vi "pmt demultiplexer control.vi"() -> ()   [LabVIEW 2017]
doc: "This example performs writes and reads on a serial port, as directed by the user. You can press the Write and Read buttons, and change the Read Count, while the example is running.\n\nThe parameters set for the serial port must match the parameters of the connected instrument or device. In this example, the Read Count parameter specifies the number of bytes that the serial port reads. If there were more bytes at the port than the specified number, those bytes would not be read. If there were less bytes at the port than the specified number, you would receive a timeout error.\n\nThis example expands upon the flow control options for XON and XOFF, allowing the user to choose those control characters. Also, the user can enable or disable a termination character. Some devices require a termination character in order to identify the end of command strings. Some devices send a termination character to signify the end of data to be read. This example shows how you can end the Read operation once a termination character is detected in the buffer and/or append a termination character at the end of the Write data."
uses:
  pmt demultiplexer command set.ctl
  <vilib>/Instr/_visa.llb/VISA Configure Serial Port (Instr).vi
panel:
  in  "encode photons as level changes":bool
  out "cross talk":dbl
  in  "dead count rate":dbl format="%#_13g"
  out "beam 2 rate":dbl
  out "beam 1 rate":dbl
  out "lock problem":bool
  in  "test input":enum8{"none", "internal", "external"}(ring)
  in  "laser cycles to veto":u8=2
  in  "start2 - start1":u16=180 step=5
  in  "width2":u16=170 max=180 step=5
  in  "width1":u16=170 max=180 step=5
  in  "auto step phase":bool
  out "version":u8[](array[numeric])
  out "cts vs phase shift":cluster{dbl[], dbl[]}[](graph)
  out "tau":dbl=0.6896638311807903
  out "dead counts":dbl=52664.79325691533
  out "exponential fit parameters":cluster{"t0":dbl, "amplitude":dbl}[](array[cluster])=[{"t0"=3.645795108508593, "amplitude"=683172.1393034825}]
  in  "timeout (ms)":i32=1000
  in  "num exp":i32=1
  out "total count rate":dbl=683172.1393034825
  out "hist data received":bool=TRUE
  out "histogram":cluster{i32[], dbl[]}[](graph)
  out "all data received":bool=TRUE
  out "response":u8[](array[numeric])
  in  "Command":T1
  in  "overall phase shift (deg)":u16=95 step=5
  out "error out":errorcluster
  in  "Stop":bool
  in  "data":u8
  in  "Send command":bool
  in  "VISA resource name":refnum<visa-resource-name>="COM8"
  # "5 deg = 200 ps @ 70 MHz"
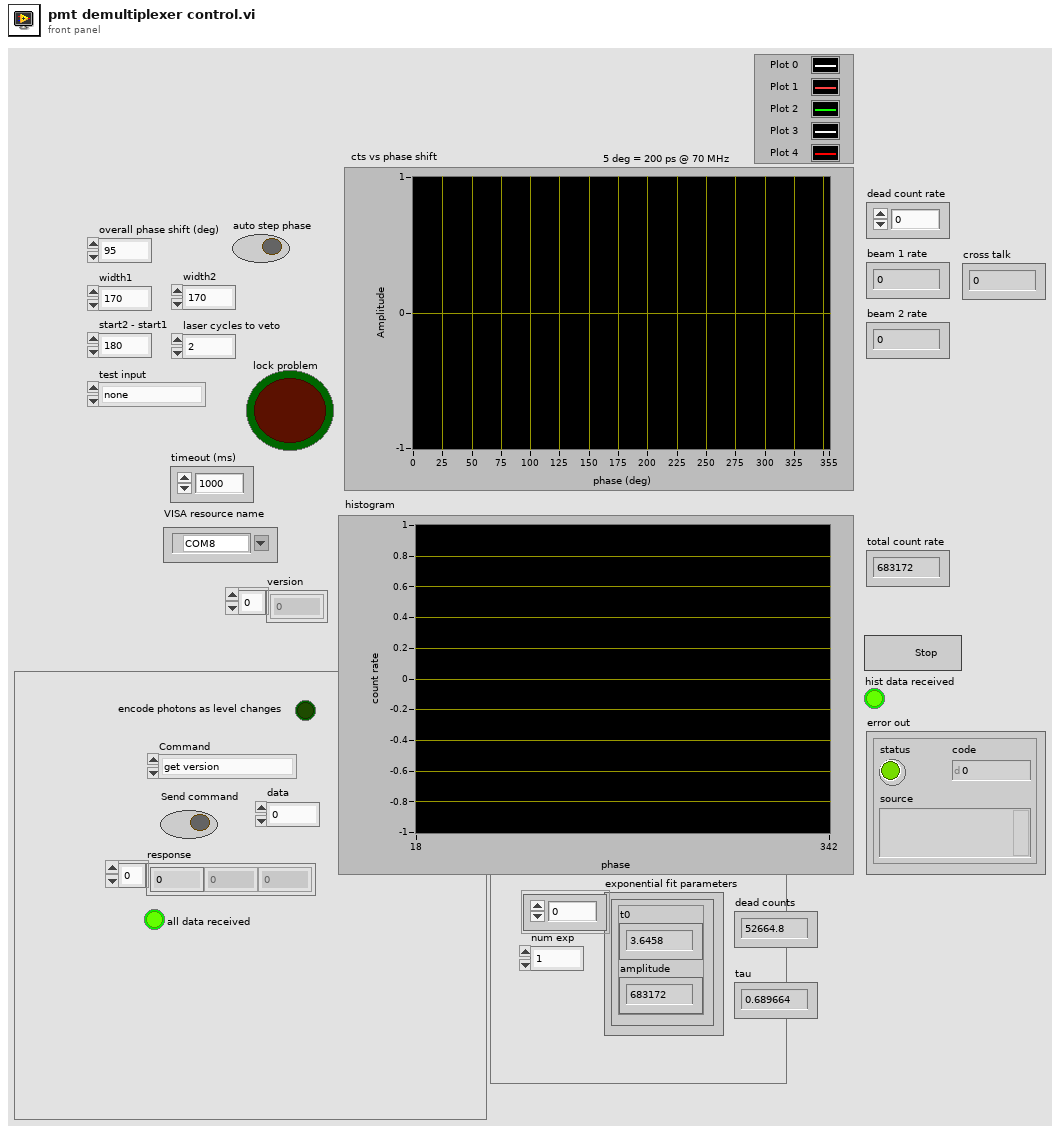
[diagram p1: front panel]
types:
  T1 = typedef "pmt demultiplexer command set.ctl" = enum8{"get version", "set outputs", "set pll", "set passthrough", "get histogram", "set pmt veto", "reset pll", "set test inputs", "get error", "encode as shift"}
  T2 = cluster{"baud rate":u32, "data bits":u16, "parity":enum16{"None", "Odd", "Even", "Mark", "Space"}, "stop bits":u16}
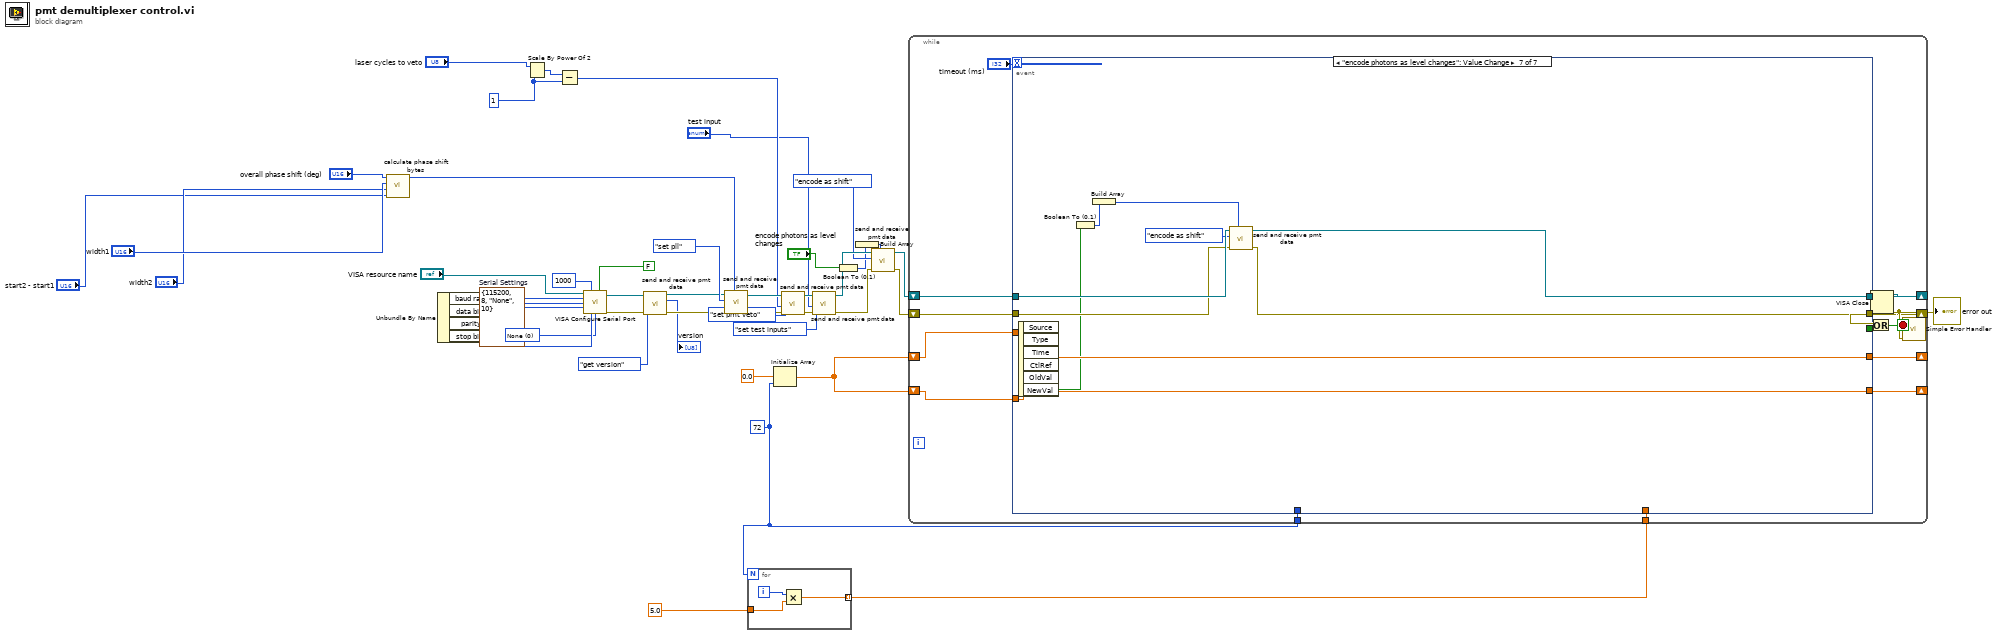
[diagram p0: block diagram]
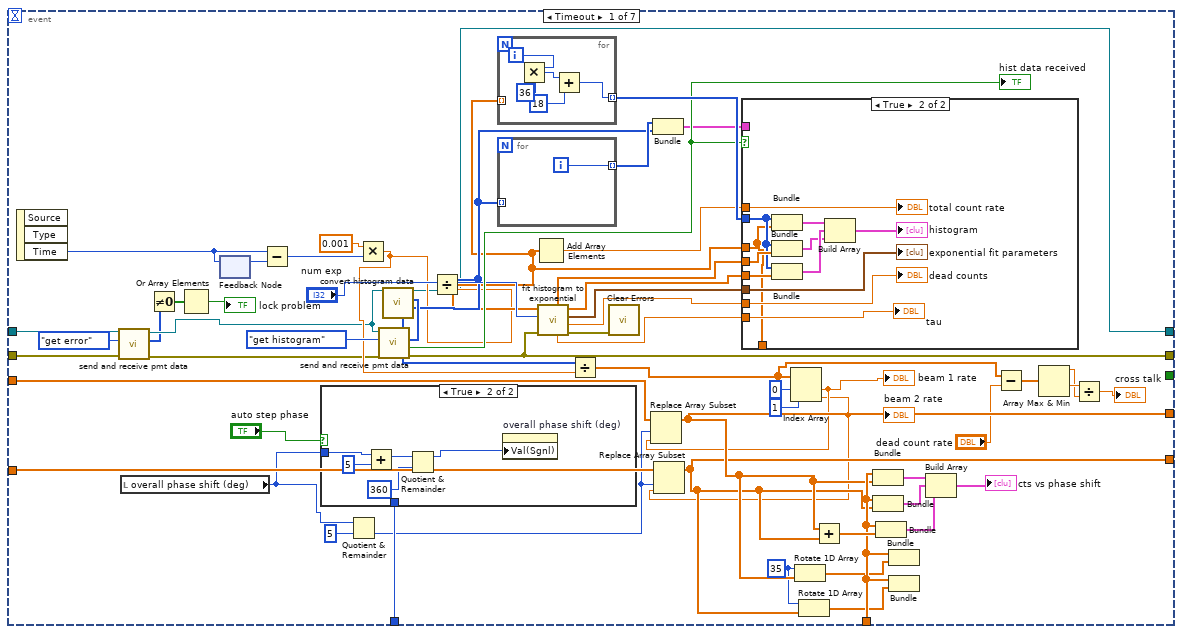
[diagram p2: hidden frame]
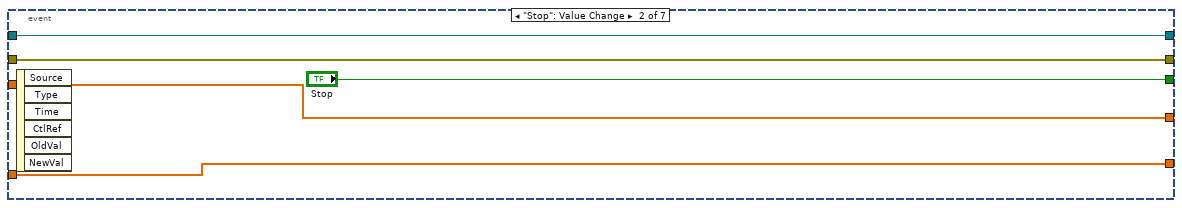
[diagram p5: hidden frame]
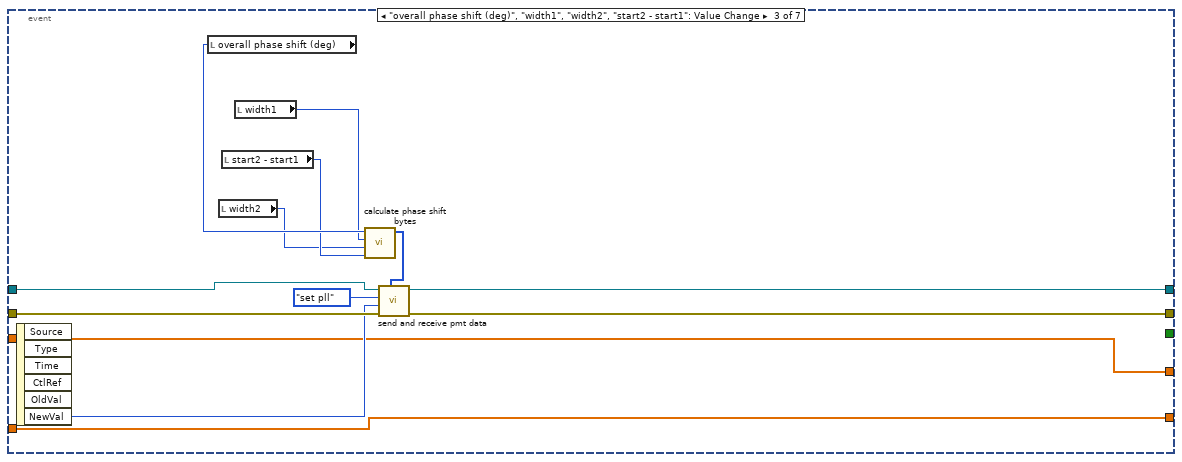
[diagram p6: hidden frame]
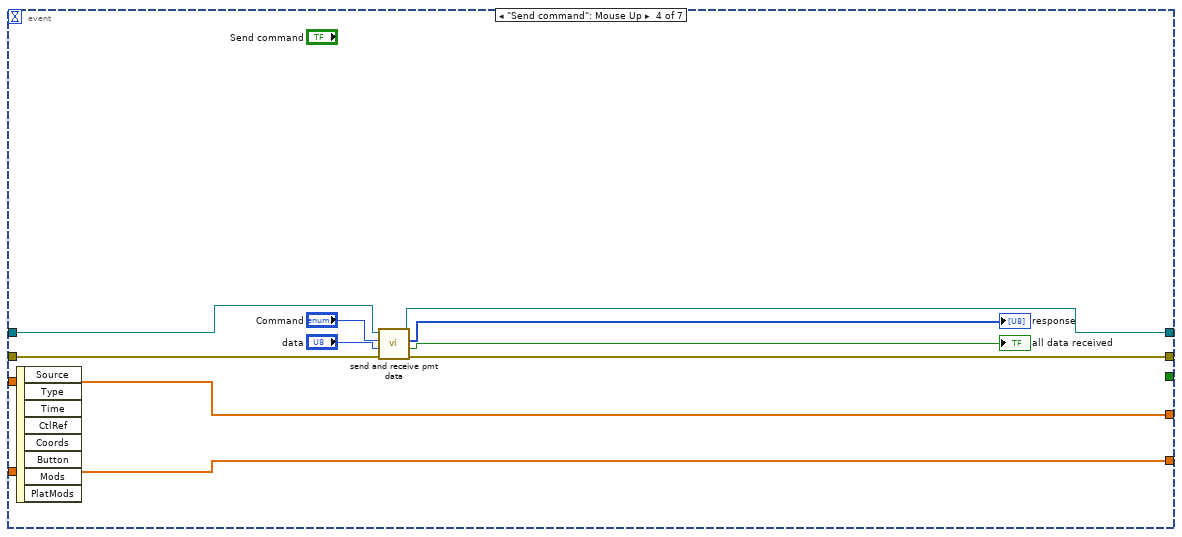
[diagram p7: hidden frame]
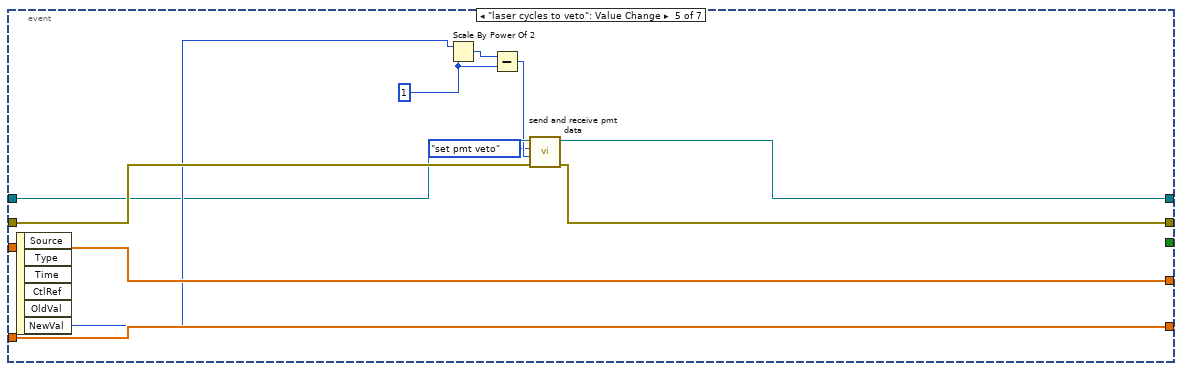
[diagram p8: hidden frame]
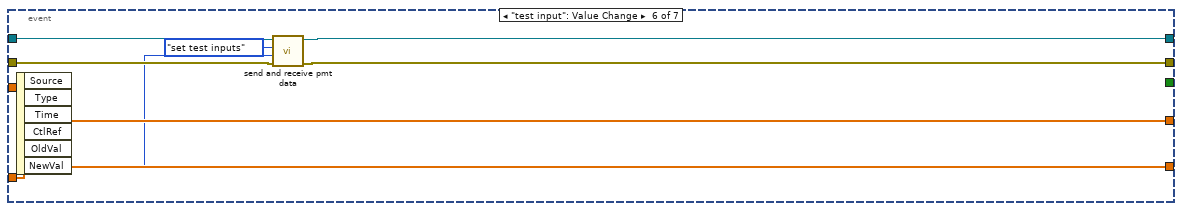
[diagram p9: hidden frame]
diagram:
  w17 = u8 1
  w27 = u8 72 ("y")
  w42 = u16 0 items=["None", "XON/XOFF", "RTS/CTS", "XON/XOFF & RTS/CTS", "DTR/DSR", "XON/XOFF & DTR/DSR"] ("flow control (0:none)")
  w43 = T2 {"baud rate"=115200, "data bits"=8, "parity"=enum."None", "stop bits"=10}  # Serial Settings
  n1 = call "calculate phase shift bytes.vi"("start2 - start1"="start2 - start1", "width2"="width2", "width1"="width1", "overall phase shift (deg)"="overall phase shift (deg)") -> ("phase shifts"=w20:u8[])  [unwired: 7 in]
  n2 = Unbundle By Name(w43) -> ("baud rate"=w44:u32, "data bits"=w45:u16, "parity"=w46:enum16{"None", "Odd", "Even", "Mark", "Space"}, "stop bits"=w47:u16)
  n3 = Scale By Power Of 2(n="laser cycles to veto", x=w17) -> (x*2^n=w18:u8)
  n4 = Subtract(x=w18, y=w17) -> (x-y=w13:u8)
  n5 = call-poly "VISA Configure Serial Port"("VISA resource name"="VISA resource name", "timeout (10sec)"=u32 1000, "Enable Termination\nChar (T)"=FALSE ("Enable Termination\nChar (T)"), "baud rate (9600)"=w44, "data bits (8)"=w45, "parity (0:none)"=w46, "stop bits (10: 1 bit)"=w47, "flow control (0:none)"=w42) -> ("VISA resource name out"=w32:refnum<visa-resource-name>, "error out"=w35:errorcluster)  [unwired: 2 in, 4 out]
  n6 = call "send and receive pmt data.vi"("error in (no error)"=w35, "Command"=pmt_demultiplexer_command_set."get version", "VISA resource"=w32) -> ("error out"=w34:errorcluster, "data out"=→"version":u8[], "visa out"=w33:refnum<visa-resource-name>)  [unwired: 5 in, 1 out]
  n7 = call "send and receive pmt data.vi"("data (byte array)"=w20, "error in (no error)"=w34, "Command"=pmt_demultiplexer_command_set."set pll", "VISA resource"=w33) -> ("error out"=w16:errorcluster, "visa out"=w15:refnum<visa-resource-name>)  [unwired: 4 in, 2 out]
  n8 = for {
    N: w27 -> [_]
    tunnel: 5.0 ("y") -> [w50]
    tunnel: [w49] -> w25 mode=indexing
    i -> [w51]
    n9 = Multiply(x=w51, y=w50) -> (x*y=w49:dbl)
  }
  n10 = Initialize Array(0.0 ("dimension size"), w27) -> (w28:dbl[])
  n11 = call "send and receive pmt data.vi"("error in (no error)"=w16, "data (byte)"=w13, "Command"=pmt_demultiplexer_command_set."set pmt veto", "VISA resource"=w15) -> ("error out"=w12:errorcluster, "visa out"=w11:refnum<visa-resource-name>)  [unwired: 4 in, 2 out]
  n12 = call "send and receive pmt data.vi"("error in (no error)"=w12, "data (byte)"="test input", "Command"=pmt_demultiplexer_command_set."set test inputs", "VISA resource"=w11) -> ("error out"=w7:errorcluster, "visa out"=w8:refnum<visa-resource-name>)  [unwired: 4 in, 2 out]
  n13 = Boolean To (0,1)(Boolean="encode photons as level changes") -> (0, 1=w2:i16)
  n14 = Build Array(w2) -> (w1:i16[])
  n15 = call "send and receive pmt data.vi"("data (byte array)"=w1, "error in (no error)"=w7, "Command"=pmt_demultiplexer_command_set."encode as shift", "VISA resource"=w8) -> ("error out"=w6:errorcluster, "visa out"=w5:refnum<visa-resource-name>)  [unwired: 4 in, 2 out]
  n16 = while {
    shift-right: [w62] -> w40
    shift-left: w5 -> [w64]
    shift-right: [w59] -> w38
    shift-left: w6 -> [w63]
    tunnel: w27 -> [w57]
    shift-right: [w55] -> _
    shift-left: w28 -> [w56]
    shift-right: [w53] -> _
    shift-left: w28 -> [w54]
    tunnel: w25 -> [w52]
    stop <- w60 stop-if-true
    n17 = event shown="[6] \"encode photons as level changes\": Value Change" {
      selector: _ -> [_ _ _ _ _ _ _]
      dyn-events: _ -> [_ _ _ _ _ _ _]
      timeout: "timeout (ms)" -> [_ _ _ _ _ _ _]
      tunnel: w64 -> [w80 w152 w165 w175 w179 w192 w202]
      tunnel: w63 -> [w78 w151 w164 w174 w182 w190 w200]
      tunnel: [w79 w152 w161 w173 w178 w191 w198] -> w62
      tunnel: [w114 w151 w160 w172 w181 w189 w199] -> w59
      tunnel: [_ "Stop" _ _ _ _ _] -> w61
      tunnel: w57 -> [w103 _ _ _ _ _ _]
      tunnel: w56 -> [w102 w149 w159 w167 w186 w194 w204]
      tunnel: [w89 w149 w159 w167 w186 w194 w204] -> w55
      tunnel: w54 -> [w99 w148 w158 w166 w185 w193 w203]
      tunnel: [w86 w148 w158 w166 w185 w193 w203] -> w53
      tunnel: w52 -> [w90 _ _ _ _ _ _]
      event Timeout {
        w87 = 35 ("n")
        n18 = event-data() -> ("Time"=w120:u32)  [unwired: 1 in, 2 out]
        n19 = call "send and receive pmt data.vi"("error in (no error)"=w78, "Command"=pmt_demultiplexer_command_set."get error", "VISA resource"=w80) -> ("error out"=w77:errorcluster, "data out"=w75:u8[], "visa out"=w79:refnum<visa-resource-name>)  [unwired: 5 in, 1 out]
        n20 = local read "overall phase shift (deg)"() -> (w84:u16)
        n21 = Not Equal To 0?(x=w75) -> (x != 0?=w74:bool[])
        n22 = Or Array Elements(Boolean array=w74) -> (logical OR=→"lock problem":bool)
        n23 = feedback-in #1(w120) -> ()
        n24 = feedback #1() -> (w119:u32)  [unwired: 1 in]
        n25 = Subtract(x=w120, y=w119) -> (x-y=w118:u32)
        n26 = case shown="True" "auto step phase" {
          tunnel: w84 -> [_ w128]
          tunnel: w103 -> [_ _]
          frame False {
          }
          frame True {
            n27 = Add(x=w128, y=u16 5) -> (x+y=w126:u16)
            n28 = Quotient & Remainder(x=w126, y=u16 360) -> (x-y*floor(x/y)=w124:u16)  [unwired: 1 out]
            n29 = property on="overall phase shift (deg)" class="DigNum (strict)"("Val(Sgnl)"=w124) -> ()  [unwired: 2 in, 2 out]
          }
        }
        n30 = Quotient & Remainder(x=w84, y=u16 5) -> (floor(x/y)=w82:u16)  [unwired: 1 out]
        n31 = Multiply(x=0.001, y=w118) -> (x*y=w81:dbl)
        n32 = call "send and receive pmt data.vi"("error in (no error)"=w77, "Command"=pmt_demultiplexer_command_set."get histogram", "VISA resource"=w79) -> ("error out"=w114:errorcluster, "all data received"=w115:bool, "data out"=w121:u8[])  [unwired: 5 in, 1 out]
        "hist data received" <- w115
        n33 = call "convert histogram data.vi"("data out"=w121) -> ("count histogram"=w93:u32[], "detection histogram"=w91:u32[])  [unwired: 8 in, 1 out]
        n34 = Divide(x=w93, y=w81) -> (x/y=w92:dbl[])
        n35 = for {
          tunnel: w92 -> [_] mode=indexing
          tunnel: [w144] -> w122 mode=indexing
          i -> [w145]
          n36 = Multiply(x=w145, y=36) -> (x*y=w143:i32)
          n37 = Add(x=w143, y=18) -> (x+y=w144:i32)
        }
        n38 = for {
          tunnel: [w129] -> w106 mode=indexing
          tunnel: w93 -> [_] mode=indexing
          i -> [w129]
        }
        n39 = Add Array Elements(numeric array=w92) -> (sum=w116:dbl)
        n40 = call "fit histogram to exponential.vi"("error in (no error)"=w114, "num exp"="num exp", "Y"=w92) -> ("error out"=w112:errorcluster, "dead counts"=w109:dbl, "exponential fit parameters"=w110:cluster{"t0":dbl, "amplitude":dbl}[], "best nonlinear fit"=w111:dbl[], "tau"=w107:dbl, "initial guess"=w108:dbl[])  [unwired: 3 in]
        n41 = Divide(x=w91, y=w81) -> (x/y=w70:dbl[])
        n42 = call <vilib>:"Clear Errors.vi"("error in (no error)"=w112) -> ()  [unwired: 5 in, 2 out]
        n43 = Bundle(w106, "count histogram"=w93) -> (w105:cluster{i32[], "count histogram":u32[]})  [unwired: 1 in]
        n44 = case shown="True" w115 {
          tunnel: w122 -> [_ w134]
          tunnel: w92 -> [w130 w131]
          tunnel: w116 -> [_ w141]
          tunnel: w111 -> [_ w138]
          tunnel: w110 -> [_ w140]
          tunnel: w109 -> [_ w139]
          tunnel: w108 -> [_ w135]
          tunnel: w107 -> [_ w132]
          tunnel: w105 -> [_ _]
          tunnel: [w130 w131] -> _
          frame False {
          }
          frame True {
            n45 = Bundle(w134, w131) -> (w142:cluster{i32[], dbl[]})  [unwired: 1 in]
            n46 = Bundle(w134, "initial guess"=w135) -> (w133:cluster{i32[], "initial guess":dbl[]})  [unwired: 1 in]
            n47 = Bundle(w134, "best nonlinear fit"=w138) -> (w136:cluster{i32[], "best nonlinear fit":dbl[]})  [unwired: 1 in]
            n48 = Build Array(w142, w136, w133) -> (→"histogram":cluster{i32[], "initial guess":dbl[]}[])
            "total count rate" <- w141
            "exponential fit parameters" <- w140
            "dead counts" <- w139
            "tau" <- w132
          }
        }
        n49 = Index Array(array=w70, index #1=0 ("index"), index #2=1 ("index")) -> (element #1=w72:dbl, element #2=w71:dbl)
        "beam 1 rate" <- w72
        "beam 2 rate" <- w71
        n50 = Replace Array Subset(array=w102, new element=w72, index=w82) -> (w89:dbl[])
        n51 = Replace Array Subset(array=w99, new element=w71, index=w82) -> (w86:dbl[])
        n52 = Rotate 1D Array(1:w89, 2:w87) -> (0:w88:dbl[])
        n53 = Rotate 1D Array(1:w86, 2:w87) -> (0:w85:dbl[])
        n54 = Add(x=w89, y=w86) -> (x+y=w95:dbl[])
        n55 = Bundle(w90, w89) -> (w98:cluster{dbl[], dbl[]})  [unwired: 1 in]
        n56 = Bundle(w90, w86) -> (w97:cluster{dbl[], dbl[]})  [unwired: 1 in]
        n57 = Bundle(w90, w95) -> (w94:cluster{dbl[], dbl[]})  [unwired: 1 in]
        n58 = Bundle(w90, w88) -> ()  [unwired: 1 in, 1 out]
        n59 = Bundle(w90, w85) -> ()  [unwired: 1 in, 1 out]
        n60 = Build Array(w98, w97, w94) -> (→"cts vs phase shift":cluster{dbl[], dbl[]}[])
        n61 = Subtract(x=w70, y="dead count rate") -> (x-y=w68:dbl[])
        n62 = Array Max & Min(array=w68) -> (max value=w66:dbl, min value=w67:dbl)  [unwired: 2 out]
        n63 = Divide(x=w67, y=w66) -> (x/y=→"cross talk":dbl)
      }
      event "Stop": Value Change {
        n64 = event-data() -> ()  [unwired: 1 in, 6 out]
      }
      event "overall phase shift (deg)", "width1", "width2", "start2 - start1": Value Change {
        n65 = event-data() -> ("NewVal"=w162:u16)  [unwired: 1 in, 5 out]
        n66 = local read "overall phase shift (deg)"() -> (w157:u16)
        n67 = local read "width2"() -> (w154:u16)
        n68 = local read "start2 - start1"() -> (w155:u16)
        n69 = local read "width1"() -> (w156:u16)
        n70 = call "calculate phase shift bytes.vi"("start2 - start1"=w155, "width2"=w154, "width1"=w156, "overall phase shift (deg)"=w157) -> ("phase shifts"=w153:u8[])  [unwired: 7 in]
        n71 = call "send and receive pmt data.vi"("data (byte array)"=w153, "error in (no error)"=w164, "data (byte)"=w162, "Command"=pmt_demultiplexer_command_set."set pll", "VISA resource"=w165) -> ("error out"=w160:errorcluster, "visa out"=w161:refnum<visa-resource-name>)  [unwired: 3 in, 2 out]
      }
      event "Send command": Mouse Up {
        n72 = event-data() -> ()  [unwired: 1 in, 8 out]
        n73 = call "send and receive pmt data.vi"("error in (no error)"=w174, "data (byte)"="data", "Command"="Command", "VISA resource"=w175) -> ("error out"=w172:errorcluster, "all data received"=→"all data received":bool, "data out"=→"response":u8[], "visa out"=w173:refnum<visa-resource-name>)  [unwired: 4 in]
      }
      event "laser cycles to veto": Value Change {
        w183 = u8 1
        n74 = event-data() -> ("NewVal"=w180:u8)  [unwired: 1 in, 5 out]
        n75 = Scale By Power Of 2(n=w180, x=w183) -> (x*2^n=w184:u8)
        n76 = Subtract(x=w184, y=w183) -> (x-y=w177:u8)
        n77 = call "send and receive pmt data.vi"("error in (no error)"=w182, "data (byte)"=w177, "Command"=pmt_demultiplexer_command_set."set pmt veto", "VISA resource"=w179) -> ("error out"=w181:errorcluster, "visa out"=w178:refnum<visa-resource-name>)  [unwired: 4 in, 2 out]
      }
      event "test input": Value Change {
        n78 = event-data() -> ("NewVal"=w188:enum8{"none", "internal", "external"})  [unwired: 1 in, 5 out]
        n79 = call "send and receive pmt data.vi"("error in (no error)"=w190, "data (byte)"=w188, "Command"=pmt_demultiplexer_command_set."set test inputs", "VISA resource"=w192) -> ("error out"=w189:errorcluster, "visa out"=w191:refnum<visa-resource-name>)  [unwired: 4 in, 2 out]
      }
      event "encode photons as level changes": Value Change {
        n80 = event-data() -> ("NewVal"=w197:bool)  [unwired: 1 in, 5 out]
        n81 = Boolean To (0,1)(Boolean=w197) -> (0, 1=w196:i16)
        n82 = Build Array(w196) -> (w195:i16[])
        n83 = call "send and receive pmt data.vi"("data (byte array)"=w195, "error in (no error)"=w200, "Command"=pmt_demultiplexer_command_set."encode as shift", "VISA resource"=w202) -> ("error out"=w199:errorcluster, "visa out"=w198:refnum<visa-resource-name>)  [unwired: 4 in, 2 out]
      }
    }
    n84 = Or(x=w59, y=w61) -> (x .or. y?=w60:bool)
  }
  n85 = VISA Close(VISA resource name=w40, error in (no error)=w38) -> (error out=w39:errorcluster)
  "error out" <- w39
  n86 = call <vilib>:"Simple Error Handler.vi"("error in (no error)"=w39) -> ()  [unwired: 1 in, 8 out]
